vi "AFM_OverlayConfigurator.vi"(8 "Error In":errorcluster, 9 "Image Data Range (Main)":cluster{dbl, dbl}(slide)={46.98275862068965, 0.0} scale=0.0..100.0, 11 "Main Image (IBW)":path) -> (0 "Error Out":errorcluster)   [LabVIEW 2019]
uses:
  <vilib>/vision/Image Controls.llb/IMAQ Image.ctl
  <vilib>/JDP Science/JSONtext/JSONtext.lvlib
panel:
  out "Background out":T1
  in  "Tab Control":enum32{"App", "Documentation"}(tab)
  in  "Load Images":bool
  in  "Exit":bool
  in  "Overlay Image (IBW)":path
  out "Inkscape Config":T2 {"Width/Height" format="%#_6p"; "Y Pos" format="%#_6p"; "X Pos" format="%#_6p"}
  out "Render (Main)":T1(plugin-control)
  in  "Save Overlay":bool
  out "Render (Overlay)":T1(plugin-control)
  in  "Image Data Range (Overlay)":cluster{dbl, dbl}(slide)={46.98275862068965, 0.0} scale=0.0..100.0
  # "AFM Image Overlay Configurator"
  # "This program helps you to overlay/align two AFM background images in Inkscape. Usually this is used when the user needs to overlay a smaller HighRes scan with a \nLarger LowRes scan in Inkscape to design their devices with reference to a smaller feature on the sample.\n\nOperation:\n1. Open the path of your Main Scan (IBW)\n2. Open the path of your Reference (Overlay) Image (IBW)\n3. Click Load- This will:\n         i) Give you a preview of the two images\n         ii) Give you the Inkscape Parameters of the Overlay\n\n4. Adjust the sliders to get a clear enough image\n5. Click 'Save Overlay as JPG' to save a JPG copy of your overlay\n6. Import/DragnDrop the JPG to your Main Inkscape file and input the calculated Inkscape Params for the overlay image\n\n\n\n\n\n\n\n\n\n\n\n\n\n\n\n\nAuthored by Pubudu W."
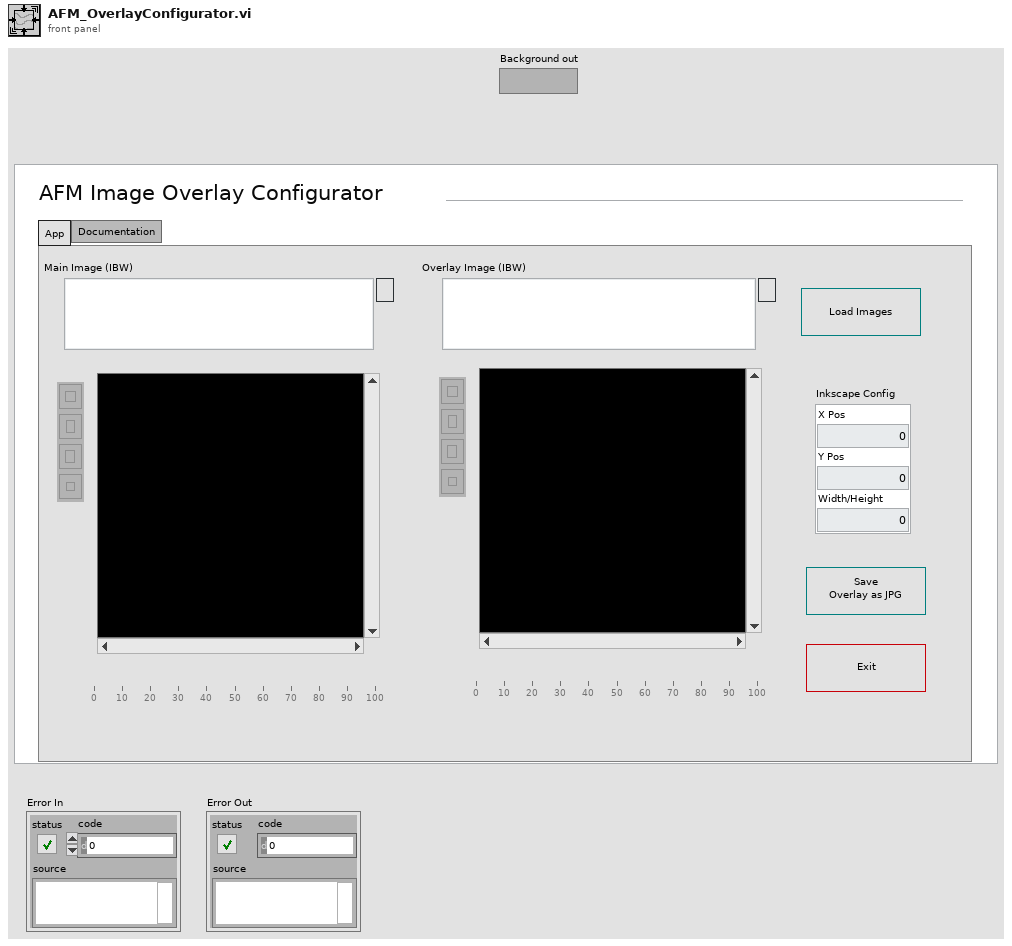
[diagram p1: front panel]
types:
  T1 = typedef "IMAQ Image.ctl" = refnum<image>
  T2 = cluster{"X Pos":dbl, "Y Pos":dbl, "Width/Height":dbl}
  T3 = enum32{"Invalid", "Standard", "Closed", "Hidden", "Minimized", "Maximized"}
  T4 = enum32{"invalid app kind", "Development System", "Run Time System", "Student Edition", "Embedded LabVIEW", "Evaluation", "Custom"}
  T5 = cluster{"Core":cluster{"Current VI Reference":refnum<vi>, "Close Panel on Exit?":bool}, "Main Image Params":cluster{"Initial ScanSize":string, "Initial XOffset":string, "Initial YOffset":string}, "Overlay Image Params":cluster{"Initial ScanSize":string, "Initial XOffset":string, "Initial YOffset":string}}
  T6 = cluster{"Initial ScanSize":string, "Initial XOffset":string, "Initial YOffset":string}
  T7 = cluster{"Current VI Reference":refnum<vi>, "Close Panel on Exit?":bool}
  T8 = typedef "Image Type" = u32
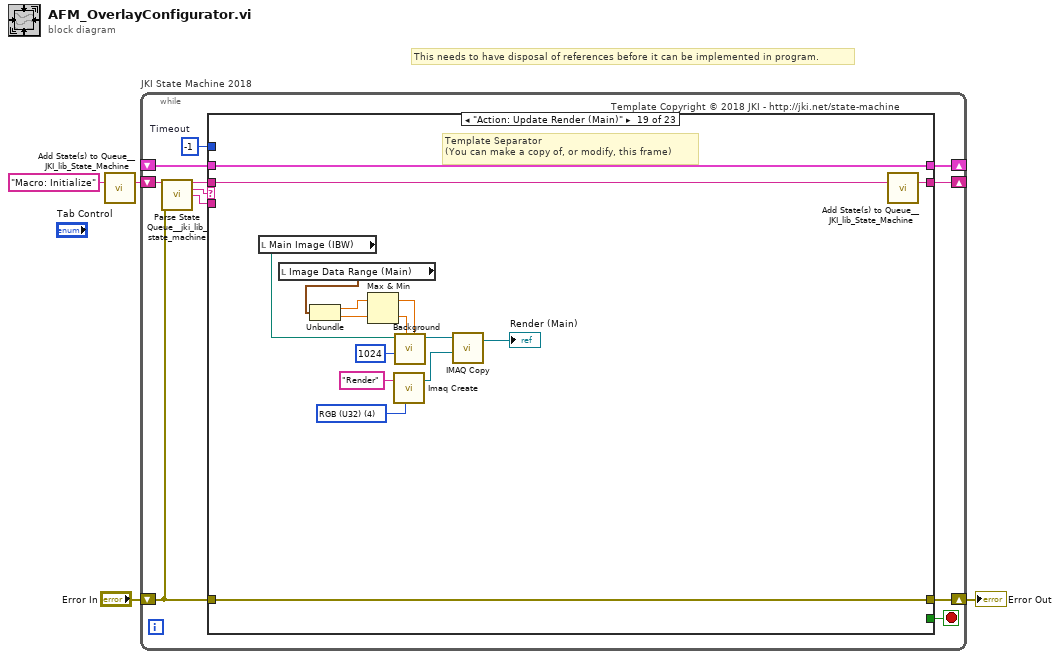
[diagram p0: block diagram]
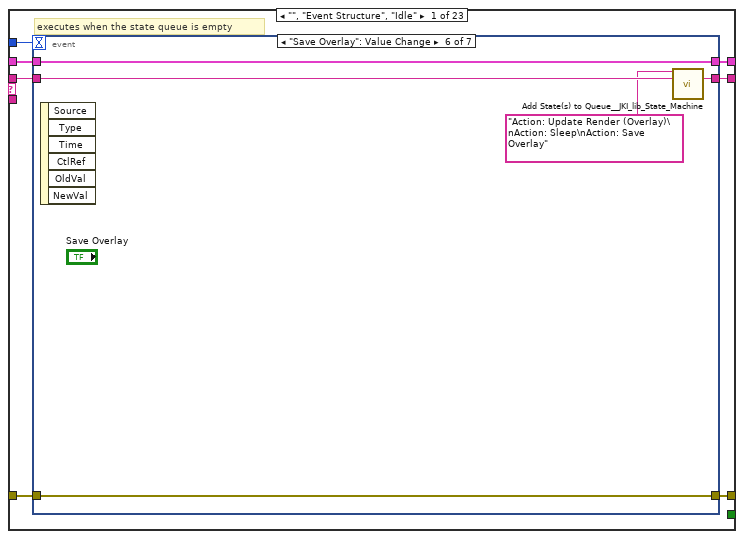
[diagram p2: hidden frame]
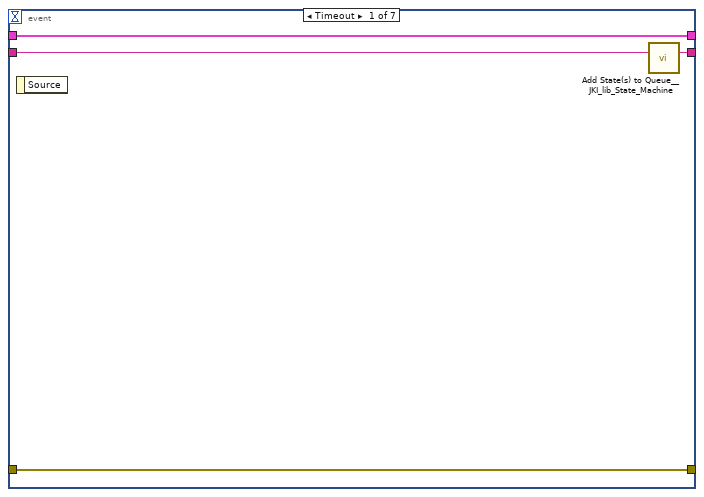
[diagram p3: hidden frame]
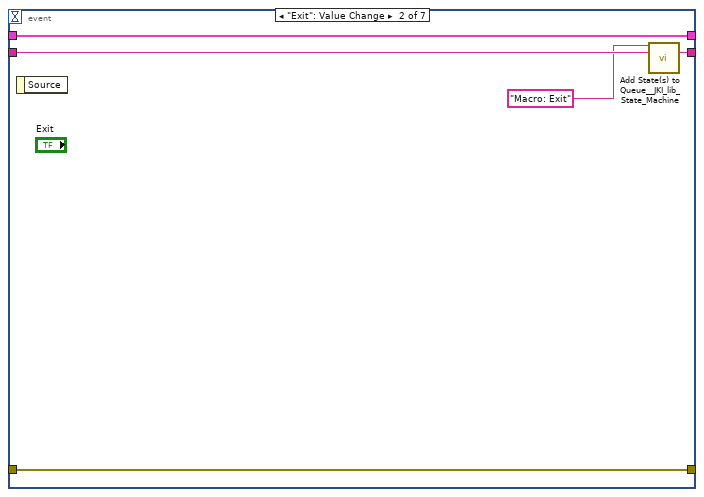
[diagram p4: hidden frame]
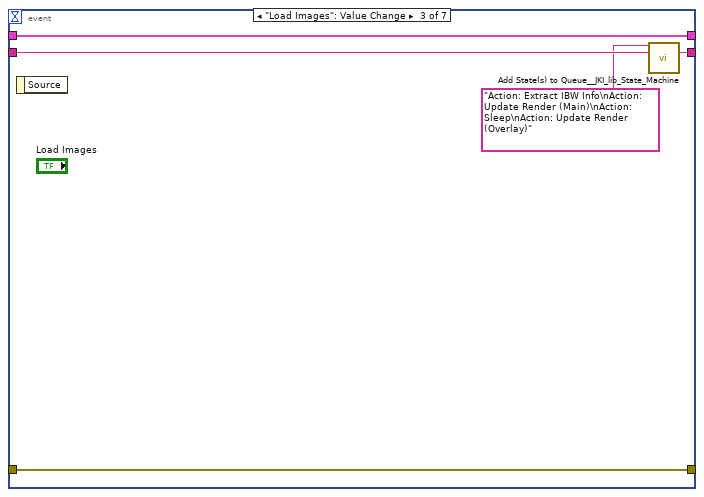
[diagram p5: hidden frame]
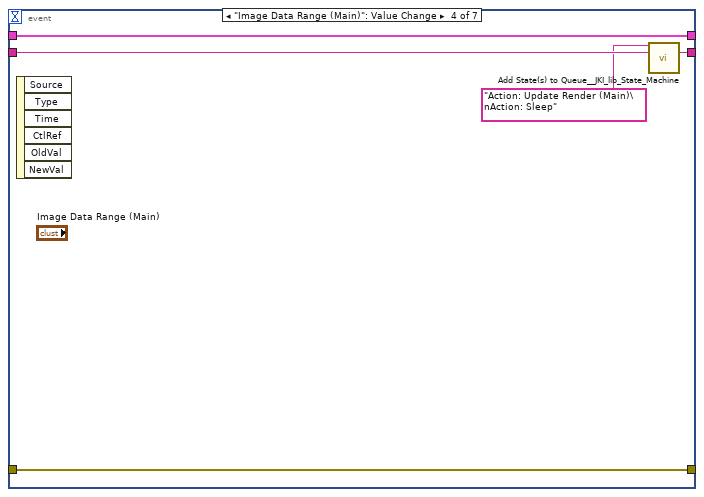
[diagram p6: hidden frame]
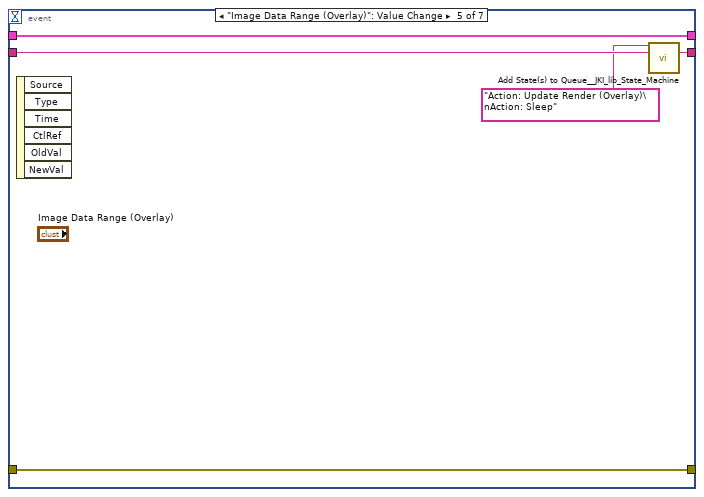
[diagram p7: hidden frame]
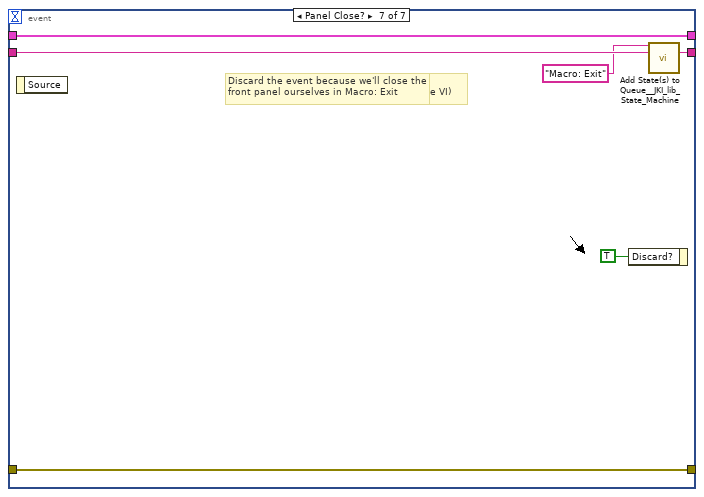
[diagram p8: hidden frame]
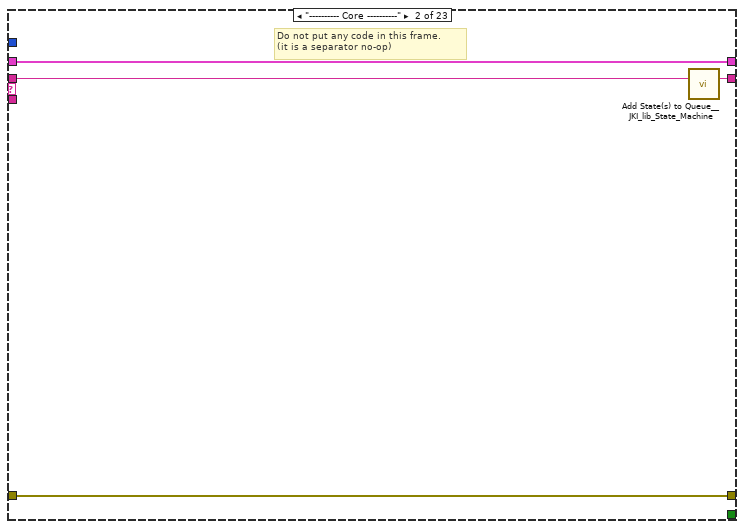
[diagram p9: hidden frame]
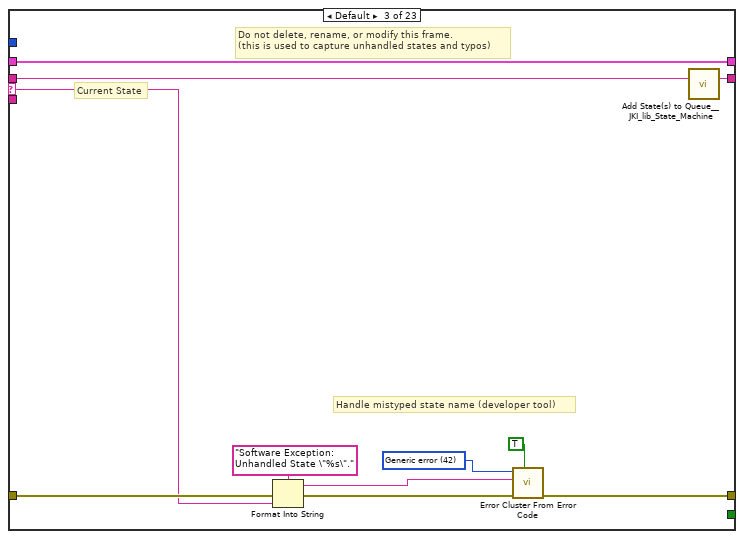
[diagram p10: hidden frame]
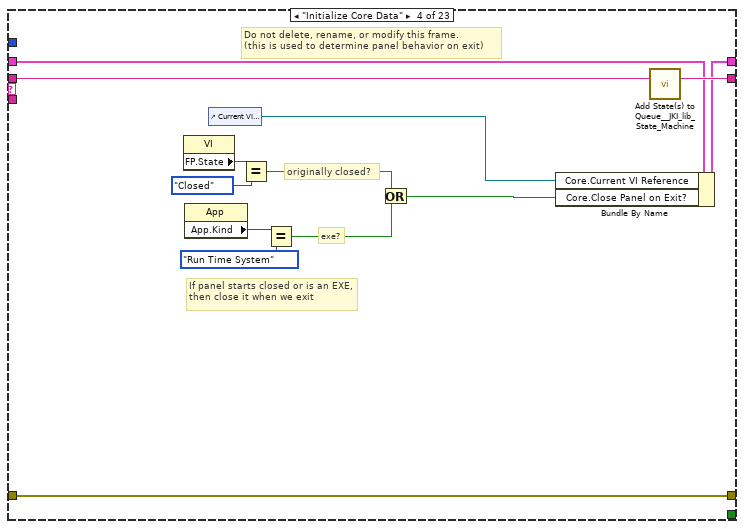
[diagram p11: hidden frame]
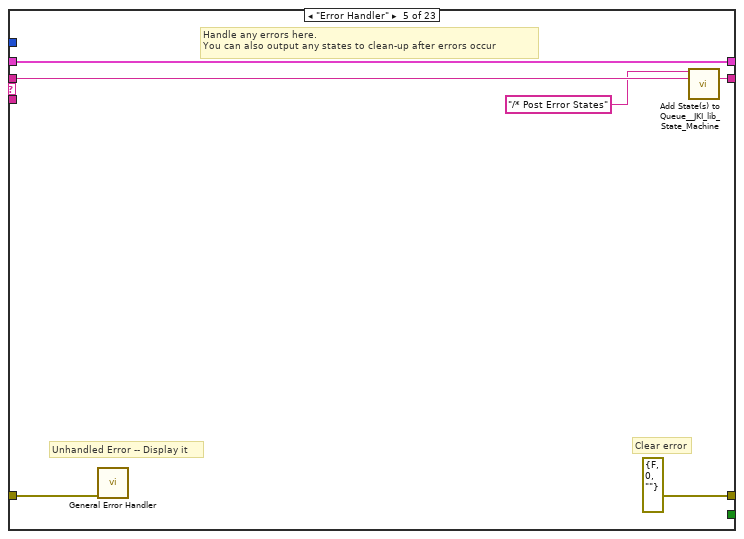
[diagram p12: hidden frame]
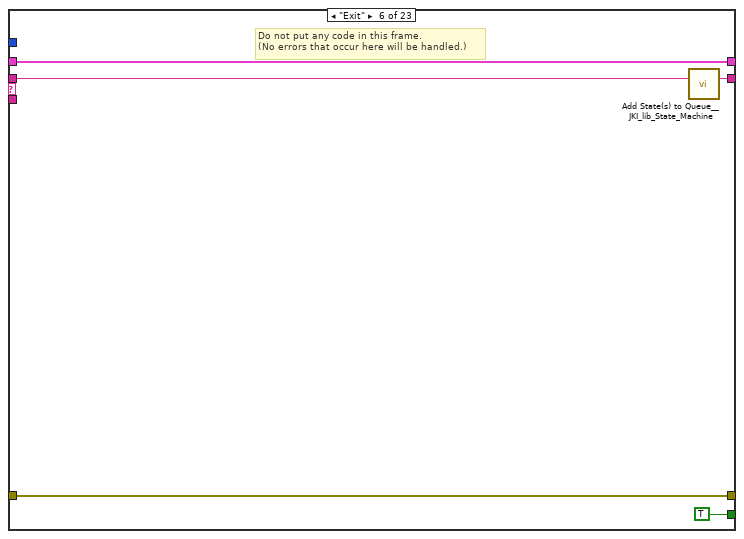
[diagram p13: hidden frame]
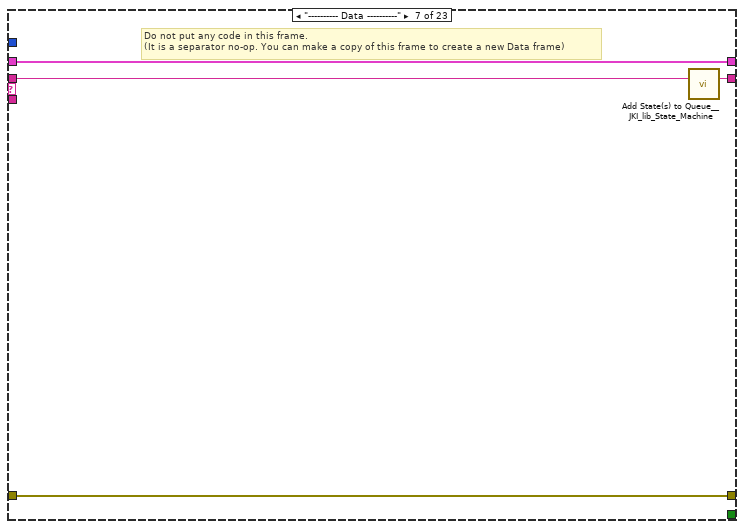
[diagram p14: hidden frame]
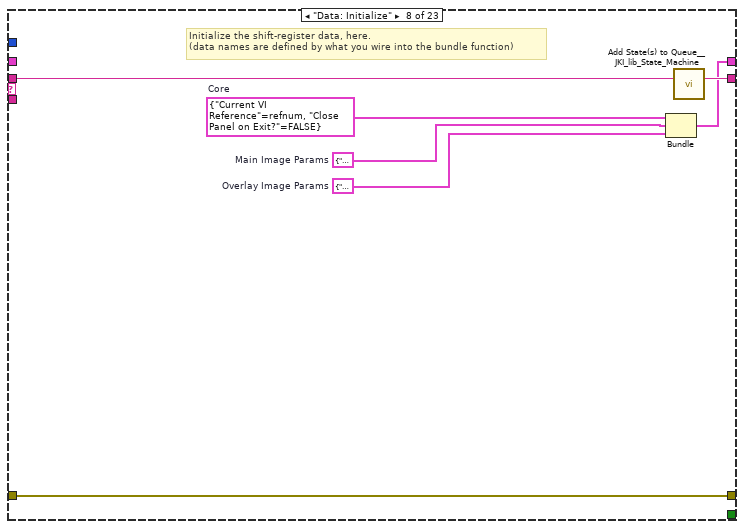
[diagram p15: hidden frame]
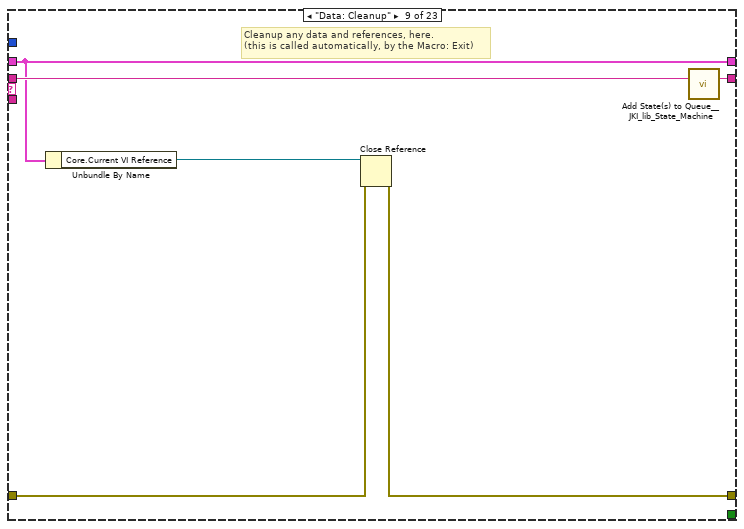
[diagram p16: hidden frame]
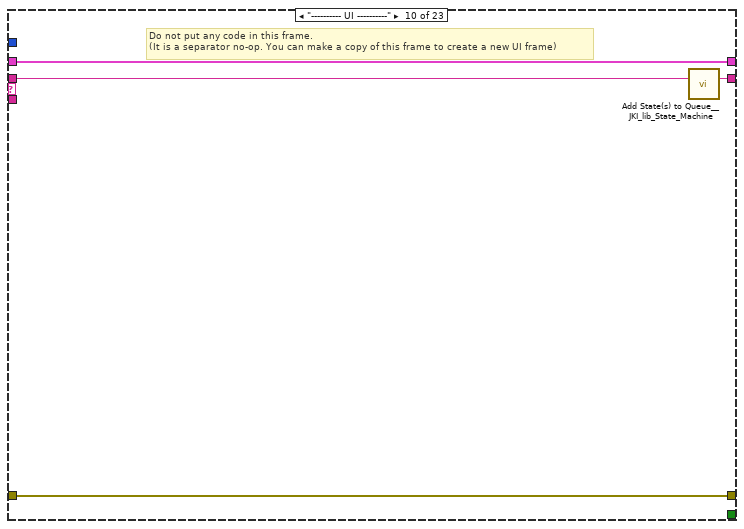
[diagram p17: hidden frame]
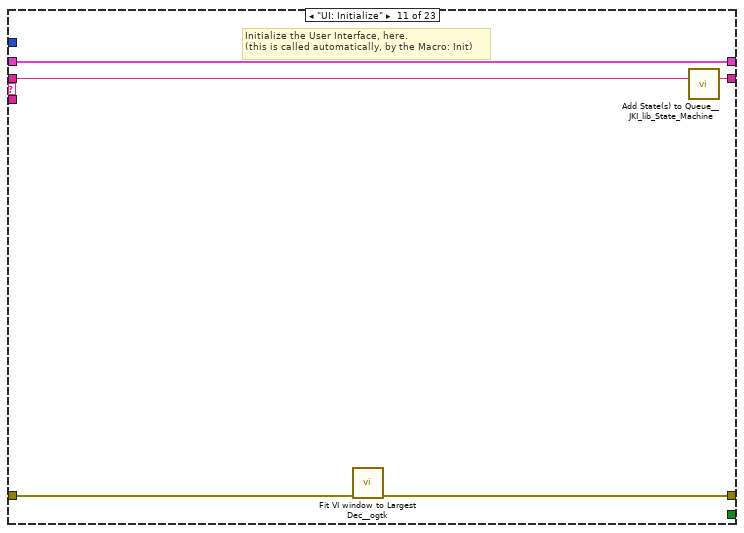
[diagram p18: hidden frame]
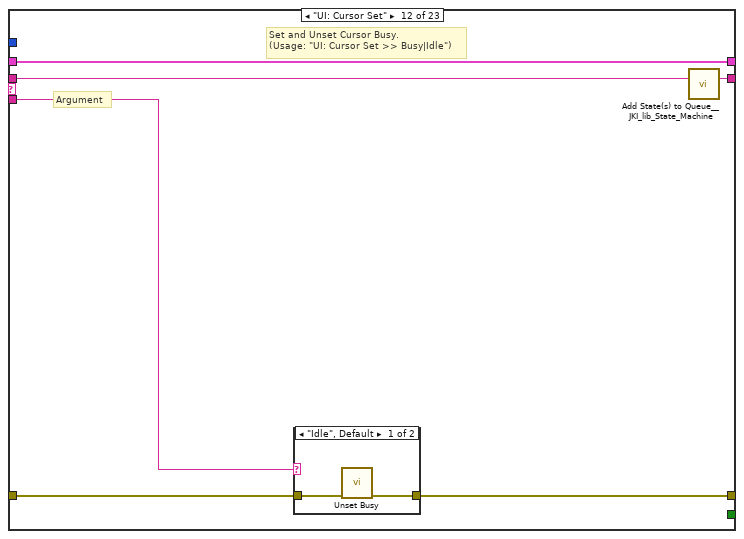
[diagram p19: hidden frame]
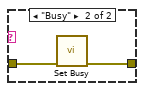
[diagram p20: hidden frame]
diagram:
  # "This needs to have disposal of references before it can be implemented in program."
  n1 = call <vilib>:"Add State(s) to Queue__JKI_lib_State_Machine.vi"("State(s) in (\"\")"="Macro: Initialize") -> ("States Out"=w4:string)  [unwired: 14 in]
  n2 = while "JKI State Machine 2018" {
    shift-right: [w8] -> _
    shift-left: _ -> [w7]
    shift-right: [w11] -> w1
    shift-left: "Error In" -> [w5]
    shift-right: [w10] -> _
    shift-left: w4 -> [w12]
    stop <- w9 stop-if-true
    w6 = -1  # Timeout
    # "Template Copyright © 2018 JKI - http://jki.net/state-machine"
    n3 = call <vilib>:"Parse State Queue__jki_lib_state_machine.vi"("State Queue"=w12, "Error In (no error)"=w5) -> ("Remaining States"=w14:string, "Current State"=w15:string, "Arguments"=w13:string)  [unwired: 11 in]
    n4 = case shown="\"Action: Update Render (Main)\"" w15 {
      selector: w15 -> [_ _ w62 _ _ _ _ _ _ _ _ _ _ _ _ _ _ _ _ _ _ _ _]
      tunnel: w14 -> [w22 w61 w66 w85 w91 w96 w100 w107 w113 w117 w122 w128 w139 w208 w213 w223 w227 w246 w262 w278 w284 w297 w324]
      tunnel: w13 -> [_ _ _ _ _ _ _ _ _ _ _ w123 w133 _ _ _ _ _ _ _ _ _ _]
      tunnel: w7 -> [w20 w58 w64 w78 w88 w94 w97 _ w108 w114 w120 w126 w135 w205 w210 w220 w224 w233 w259 w275 w282 w295 w321]
      tunnel: [w19 w59 w68 w82 errorcluster {"status"=FALSE, "code"=0, "source"=""} ("error out") w93 w98 w104 w109 w115 w119 w124 w136 w206 w211 w221 w225 w235 w260 w276 w279 w285 w322] -> w11
      tunnel: w5 -> [w18 w59 w67 w82 w87 w93 w98 w104 w110 w115 w118 w125 w137 w206 w211 w221 w225 w243 w260 w276 w280 w287 w322]
      tunnel: [w21 w60 w65 w84 w90 w95 w99 w106 w112 w116 w121 w127 w138 w207 w212 w222 w226 w245 w261 w277 w283 w296 w323] -> w10
      tunnel: [_ _ _ _ _ TRUE _ _ _ _ _ _ _ _ _ _ _ _ _ _ _ _ _] -> w9
      tunnel: [w17 w58 w64 w83 w88 w94 w97 w105 w108 w114 w120 w126 w135 w205 w210 w220 w224 w232 w259 w275 w282 w295 w321] -> w8
      tunnel: w6 -> [w16 _ _ _ _ _ _ _ _ _ _ _ _ _ _ _ _ _ _ _ _ _ _]
      frame "", "Event Structure", "Idle" {
        # "executes when the state queue is empty"
        n5 = event shown="[5] \"Save Overlay\": Value Change" {
          selector: _ -> [_ _ _ _ _ _ _]
          dyn-events: _ -> [_ _ _ _ _ _ _]
          timeout: w16 -> [_ _ _ _ _ _ _]
          tunnel: w22 -> [w26 w31 w36 w41 w46 w51 w57]
          tunnel: [w25 w30 w35 w40 w45 w50 w56] -> w21
          tunnel: w20 -> [w23 w28 w33 w38 w43 w48 w54]
          tunnel: [w24 w29 w34 w39 w44 w49 w55] -> w19
          tunnel: w18 -> [w24 w29 w34 w39 w44 w49 w55]
          tunnel: [w23 w28 w33 w38 w43 w48 w54] -> w17
          event Timeout {
            n6 = event-data() -> ()  [unwired: 1 in, 1 out]
            n7 = call <vilib>:"Add State(s) to Queue__JKI_lib_State_Machine.vi"("State(s) in (\"\")"=w26) -> ("States Out"=w25:string)  [unwired: 14 in]
          }
          event "Exit": Value Change {
            n8 = event-data() -> ()  [unwired: 1 in, 1 out]
            n9 = call <vilib>:"Add State(s) to Queue__JKI_lib_State_Machine.vi"("State(s) in Front (\"\")"="Macro: Exit", "State(s) in (\"\")"=w31) -> ("States Out"=w30:string)  [unwired: 13 in]
          }
          event "Load Images": Value Change {
            n10 = event-data() -> ()  [unwired: 1 in, 1 out]
            n11 = call <vilib>:"Add State(s) to Queue__JKI_lib_State_Machine.vi"("State(s) in Front (\"\")"="Action: Extract IBW Info\nAction: Update Render (Main)\nAction: Sleep\nAction: Update Render (Overlay)", "State(s) in (\"\")"=w36) -> ("States Out"=w35:string)  [unwired: 13 in]
          }
          event "Image Data Range (Main)": Value Change {
            n12 = event-data() -> ()  [unwired: 1 in, 6 out]
            n13 = call <vilib>:"Add State(s) to Queue__JKI_lib_State_Machine.vi"("State(s) in Front (\"\")"="Action: Update Render (Main)\nAction: Sleep", "State(s) in (\"\")"=w41) -> ("States Out"=w40:string)  [unwired: 13 in]
          }
          event "Image Data Range (Overlay)": Value Change {
            n14 = event-data() -> ()  [unwired: 1 in, 6 out]
            n15 = call <vilib>:"Add State(s) to Queue__JKI_lib_State_Machine.vi"("State(s) in Front (\"\")"="Action: Update Render (Overlay)\nAction: Sleep", "State(s) in (\"\")"=w46) -> ("States Out"=w45:string)  [unwired: 13 in]
          }
          event "Save Overlay": Value Change {
            n16 = event-data() -> ()  [unwired: 1 in, 6 out]
            n17 = call <vilib>:"Add State(s) to Queue__JKI_lib_State_Machine.vi"("State(s) in Front (\"\")"="Action: Update Render (Overlay)\nAction: Sleep\nAction: Save Overlay", "State(s) in (\"\")"=w51) -> ("States Out"=w50:string)  [unwired: 13 in]
          }
          event Panel Close? {
            # "Discard the event because we'll close the front panel ourselves in Macro: Exit"
            # "Close Panel button (pressed) Event\n(this executes Macro: Exit to terminate the VI)"
            n18 = event-data() -> ()  [unwired: 1 in, 1 out]
            n19 = event-data("Discard?"=TRUE) -> ()  [unwired: 1 in, 1 out]
            n20 = call <vilib>:"Add State(s) to Queue__JKI_lib_State_Machine.vi"("State(s) in Front (\"\")"="Macro: Exit", "State(s) in (\"\")"=w57) -> ("States Out"=w56:string)  [unwired: 13 in]
          }
        }
      }
      frame "---------- Core ----------" {
        # "Do not put any code in this frame.\n(it is a separator no-op)"
        n21 = call <vilib>:"Add State(s) to Queue__JKI_lib_State_Machine.vi"("State(s) in (\"\")"=w61) -> ("States Out"=w60:string)  [unwired: 14 in]
      }
      frame Default {
        w71 = 42 items=["No error", "Argument error", "Memory is full", "Out of zone", "End of file", "File already open", "Generic file I/O error", "File not found", "File permission error", "Disk is full", "Duplicate path", "Too many files open", "System feature not enabled", "Resource file not found", "Cannot add resource", "Resource not found", "Image not found", "Image memory error", "Pen does not exist", "Config type invalid", "Config token not found", "Config parse error", "Config memory error", "Bad external code format", "Bad external code offset", "External code not present", "Null window", "Destroy window error", "Null menu", "Print aborted", "Bad print record", "Print driver error", "Windows error during printing", "Memory error during printing", "Print dialog error", "Generic print error", "Invalid device refnum", "Device not found", "Device parameter error", "Device unit error", "Cannot open device", "Device call aborted", "Generic error", "Cancelled by user", "Object ID too low", "Object ID too high", "Object not in heap", "Unknown heap", "Unknown object (invalid DefProc)", "Unknown object (DefProc not in table)", "Message out of range", "Invalid (null) method", "Unknown message", "Manager call not supported", "Bad address", "Network operation in progress", "Network operation timed out", "Connection is busy", "Network attribute not supported", "Network error", "Address in use", "System out of memory", "Connection aborted", "Connection refused", "Not connected", "Already connected", "Connection closed", "Initialization error (interapplication manager)", "Bad occurrence", "Wait on unbound occurrence handler", "Occurrence queue overflow", "Datalog type conflict", "Unused", "Unrecognized type (interapplication manager)", "Memory corrupt", "Failed to make temporary DLL", "Old CIN version", "Drag socket not found", "Failed to load drop-object", "Failed to register OLE object", "Failed to release OLE object", "Format specifier type mismatch", "Unknown format specifier", "Too few format specifiers", "Too many format specifiers", "Scan failed", "Newer CIN version", "Error converting to variant", "Runtime menu error", "Password tampered", "Variant attribute not found", "Incompatible variant data type", "Event data is not available", "Event Store is not present", "Occurrence is not found", "Event Queue is not created", "Event info is not available", "Refnum passed is NULL", "Error retrieving Class GUID", "Error retrieving CoClass GUID", "Error retrieving TypeLib GUID.", "Bad built application magic bytes.", "Specific driver is different from the specific driver associated with the Logical Name.", "There is no session opened to the class driver.", "Max Error", "MAX - Error with config objects", "MAX - Error loading configuration", "MAX - Group not supported"]
        # "Current State"
        # "Do not delete, rename, or modify this frame.\n(this is used to capture unhandled states and typos)"
        # "Handle mistyped state name (developer tool)"
        n22 = Format Into String(format string="Software Exception: Unhandled State \"%s\"." ("message"), error in=w67, w62) -> (resulting string=w70:string, error out=w69:errorcluster)  [unwired: 1 in]
        n23 = call <vilib>:"Error Cluster From Error Code.vi"("show call chain? (False)"=TRUE, "error in (no error)"=w69, "error message (\"\")"=w70, "error code (0)"=w71) -> ("error out"=w68:errorcluster)  [unwired: 5 in]
        n24 = call <vilib>:"Add State(s) to Queue__JKI_lib_State_Machine.vi"("State(s) in (\"\")"=w66) -> ("States Out"=w65:string)  [unwired: 14 in]
      }
      frame "Initialize Core Data" {
        # "Do not delete, rename, or modify this frame.\n(this is used to determine panel behavior on exit)"
        # "originally closed?"
        # "exe?"
        # "If panel starts closed or is an EXE, then close it when we exit"
        n25 = property class="VI"() -> ("FP.State"=w75:T3)  [unwired: 2 in, 2 out]
        n26 = property class="App"() -> ("App.Kind"=w81:T4)  [unwired: 2 in, 2 out]
        n27 = control-ref of="Current VI Reference"() -> (w76:refnum<vi>)
        n28 = Equal?(x=w75, y=T3."Closed" ("Front Panel Window:State")) -> (x = y?=w73:bool)
        n29 = Equal?(x=w81, y=T4."Run Time System" ("Application:Kind")) -> (x = y?=w79:bool)
        n30 = Or(x=w73, y=w79) -> (x .or. y?=w77:bool)
        n31 = Bundle By Name(cluster=w78, "Core.Current VI Reference"=w76, "Core.Close Panel on Exit?"=w77) -> (w83:T5)
        n32 = call <vilib>:"Add State(s) to Queue__JKI_lib_State_Machine.vi"("State(s) in (\"\")"=w85) -> ("States Out"=w84:string)  [unwired: 14 in]
      }
      frame "Error Handler" {
        # "Unhandled Error -- Display it"
        # "Handle any errors here.\nYou can also output any states to clean-up after errors occur"
        # "Clear error"
        n33 = call <vilib>:"General Error Handler.vi"("error in (no error)"=w87) -> ()  [unwired: 10 in, 5 out]
        n34 = call <vilib>:"Add State(s) to Queue__JKI_lib_State_Machine.vi"("State(s) in Front (\"\")"="/* Post Error States", "State(s) in (\"\")"=w91) -> ("States Out"=w90:string)  [unwired: 13 in]
      }
      frame "Exit" {
        # "Do not put any code in this frame.\n(No errors that occur here will be handled.)"
        n35 = call <vilib>:"Add State(s) to Queue__JKI_lib_State_Machine.vi"("State(s) in (\"\")"=w96) -> ("States Out"=w95:string)  [unwired: 14 in]
      }
      frame "---------- Data ----------" {
        # "Do not put any code in this frame.\n(It is a separator no-op. You can make a copy of this frame to create a new Data frame)"
        n36 = call <vilib>:"Add State(s) to Queue__JKI_lib_State_Machine.vi"("State(s) in (\"\")"=w100) -> ("States Out"=w99:string)  [unwired: 14 in]
      }
      frame "Data: Initialize" {
        w101 = T6 {"Initial ScanSize"="", "Initial XOffset"="", "Initial YOffset"=""}  # Overlay Image Params
        w102 = T6 {"Initial ScanSize"="", "Initial XOffset"="", "Initial YOffset"=""}  # Main Image Params
        w103 = T7 {"Current VI Reference"=refnum, "Close Panel on Exit?"=FALSE}  # Core
        # "Initialize the shift-register data, here.\n(data names are defined by what you wire into the bundle function)"
        n37 = Bundle("Core"=w103, "Main Image Params"=w102, "Overlay Image Params"=w101) -> (w105:T5)  [unwired: 1 in]
        n38 = call <vilib>:"Add State(s) to Queue__JKI_lib_State_Machine.vi"("State(s) in (\"\")"=w107) -> ("States Out"=w106:string)  [unwired: 14 in]
      }
      frame "Data: Cleanup" {
        # "Cleanup any data and references, here.\n(this is called automatically, by the Macro: Exit)"
        n39 = Unbundle By Name(w108) -> ("Core.Current VI Reference"=w111:refnum<vi>)
        n40 = Close Reference(reference=w111, error in (no error)=w110) -> (error out=w109:errorcluster)
        n41 = call <vilib>:"Add State(s) to Queue__JKI_lib_State_Machine.vi"("State(s) in (\"\")"=w113) -> ("States Out"=w112:string)  [unwired: 14 in]
      }
      frame "---------- UI ----------" {
        # "Do not put any code in this frame.\n(It is a separator no-op. You can make a copy of this frame to create a new UI frame)"
        n42 = call <vilib>:"Add State(s) to Queue__JKI_lib_State_Machine.vi"("State(s) in (\"\")"=w117) -> ("States Out"=w116:string)  [unwired: 14 in]
      }
      frame "UI: Initialize" {
        # "Initialize the User Interface, here.\n(this is called automatically, by the Macro: Init)"
        n43 = call <userlib>:"Fit VI window to Largest Dec__ogtk.vi"("error in (no error)"=w118) -> ("error out"=w119:errorcluster)  [unwired: 5 in, 1 out]
        n44 = call <vilib>:"Add State(s) to Queue__JKI_lib_State_Machine.vi"("State(s) in (\"\")"=w122) -> ("States Out"=w121:string)  [unwired: 14 in]
      }
      frame "UI: Cursor Set" {
        # "Argument"
        # "Set and Unset Cursor Busy.\n(Usage: \"UI: Cursor Set >> Busy|Idle\")"
        n45 = case shown="\"Idle\", Default" w123 {
          tunnel: w125 -> [w130 w132]
          tunnel: [w129 w131] -> w124
          frame "Idle", Default {
            n46 = call <vilib>:"Unset Busy.vi"("error in (no error)"=w130) -> ("error out"=w129:errorcluster)  [unwired: 10 in]
          }
          frame "Busy" {
            n47 = call <vilib>:"Set Busy.vi"("error in (no error)"=w132) -> ("error out"=w131:errorcluster)  [unwired: 9 in, 1 out]
          }
        }
        n48 = call <vilib>:"Add State(s) to Queue__JKI_lib_State_Machine.vi"("State(s) in (\"\")"=w128) -> ("States Out"=w127:string)  [unwired: 14 in]
      }
      frame "UI: Front Panel State" {
        # "Argument"
        # "Set Front Panel Open or Closed\n(Usage: \"UI: Front Panel State >> Open|Close\")"
        n49 = Unbundle By Name(w135) -> ("Core.Current VI Reference"=w134:refnum<vi>)
        n50 = case shown="\"Open\", \"Standard\", Default" w133 {
          tunnel: w137 -> [w145 w160 w171 w184 w197]
          tunnel: [w147 w161 w173 w186 w199] -> w136
          tunnel: w134 -> [w146 w158 w172 w185 w198]
          frame "Open", "Standard", Default {
            w140 = T3."Standard" ("State")
            n51 = property class="VI"(reference=w146, error in=w145) -> (reference out=w143:refnum<vi>, error out=w144:errorcluster, "FP.State"=w142:T3)
            n52 = Not Equal?(x=w142, y=w140) -> (x != y?=w141:bool)
            n53 = case shown="True" w141 {
              tunnel: [w151 w153] -> w147
              tunnel: w144 -> [w150 w153]
              tunnel: w143 -> [w149 _]
              tunnel: w140 -> [w148 _]
              frame True {
                n54 = invoke class="VI" method="FP.Open"(reference=w149, error in=w150, "Activate"=TRUE, "State"=w148) -> (error out=w151:errorcluster)  [unwired: 1 in, 4 out]
              }
              frame False {
              }
            }
          }
          frame "Close", "Closed" {
            n55 = property class="VI"(reference=w158, error in=w160) -> (reference out=w157:refnum<vi>, error out=w159:errorcluster, "FP.State"=w155:T3)
            n56 = Not Equal?(x=w155, y=T3."Closed" ("Front Panel Window:State")) -> (x != y?=w154:bool)
            n57 = case shown="True" w154 {
              tunnel: [w162 w165] -> w161
              tunnel: w159 -> [w162 w164]
              tunnel: w157 -> [_ w163]
              frame False {
              }
              frame True {
                n58 = invoke class="VI" method="FP.Close"(reference=w163, error in=w164) -> (error out=w165:errorcluster)  [unwired: 1 in, 2 out]
              }
            }
          }
          frame "Hidden", "Hide" {
            w166 = T3."Hidden" ("State")
            n59 = property class="VI"(reference=w172, error in=w171) -> (reference out=w169:refnum<vi>, error out=w170:errorcluster, "FP.State"=w168:T3)
            n60 = Not Equal?(x=w168, y=w166) -> (x != y?=w167:bool)
            n61 = case shown="True" w167 {
              tunnel: [w177 w178] -> w173
              tunnel: w170 -> [w176 w178]
              tunnel: w169 -> [w175 _]
              tunnel: w166 -> [w174 _]
              frame True {
                n62 = invoke class="VI" method="FP.Open"(reference=w175, error in=w176, "State"=w174) -> (error out=w177:errorcluster)  [unwired: 2 in, 4 out]
              }
              frame False {
              }
            }
          }
          frame "Minimize", "Minimized" {
            w179 = T3."Minimized" ("State")
            n63 = property class="VI"(reference=w185, error in=w184) -> (reference out=w182:refnum<vi>, error out=w183:errorcluster, "FP.State"=w181:T3)
            n64 = Not Equal?(x=w181, y=w179) -> (x != y?=w180:bool)
            n65 = case shown="True" w180 {
              tunnel: [w190 w191] -> w186
              tunnel: w183 -> [w189 w191]
              tunnel: w182 -> [w188 _]
              tunnel: w179 -> [w187 _]
              frame True {
                n66 = invoke class="VI" method="FP.Open"(reference=w188, error in=w189, "State"=w187) -> (error out=w190:errorcluster)  [unwired: 2 in, 4 out]
              }
              frame False {
              }
            }
          }
          frame "Maximize", "Maximized" {
            w192 = T3."Maximized" ("State")
            n67 = property class="VI"(reference=w198, error in=w197) -> (reference out=w195:refnum<vi>, error out=w196:errorcluster, "FP.State"=w194:T3)
            n68 = Not Equal?(x=w194, y=w192) -> (x != y?=w193:bool)
            n69 = case shown="True" w193 {
              tunnel: [w203 w204] -> w199
              tunnel: w196 -> [w202 w204]
              tunnel: w195 -> [w201 _]
              tunnel: w192 -> [w200 _]
              frame True {
                n70 = invoke class="VI" method="FP.Open"(reference=w201, error in=w202, "State"=w200) -> (error out=w203:errorcluster)  [unwired: 2 in, 4 out]
              }
              frame False {
              }
            }
          }
        }
        n71 = call <vilib>:"Add State(s) to Queue__JKI_lib_State_Machine.vi"("State(s) in (\"\")"=w139) -> ("States Out"=w138:string)  [unwired: 14 in]
      }
      frame "---------- Macro ----------" {
        # "Do not put any code in this frame.\n(It is a separator no-op. You can make a copy of this frame to create a new Macro frame)"
        n72 = call <vilib>:"Add State(s) to Queue__JKI_lib_State_Machine.vi"("State(s) in (\"\")"=w208) -> ("States Out"=w207:string)  [unwired: 14 in]
      }
      frame "Macro: Initialize" {
        w209 = "Data: Initialize\nInitialize Core Data\nUI: Initialize\nUI: Front Panel State >> Open"  # Data: Initialize Initialize Core Data UI: Initialize UI: Front Panel State >> Open
        # "Initialization Macro\n(This is called once, when the VI starts)"
        n73 = call <vilib>:"Add State(s) to Queue__JKI_lib_State_Machine.vi"("State(s) in Front (\"\")"=w209, "State(s) in (\"\")"=w213) -> ("States Out"=w212:string)  [unwired: 13 in]
      }
      frame "Macro: Exit" {
        # "Exit Macro\n(This is called once, when the VI exits)"
        n74 = Unbundle By Name(w220) -> ("Core.Close Panel on Exit?"=w219:bool)
        n75 = Select(t="UI: Front Panel State >> Close", s=w219, f="") -> (s? t:f=w216:string)
        n76 = call <vilib>:"Add State(s) to Queue__JKI_lib_State_Machine.vi"("State(s) in (\"\")"=w216, "State(s) at Back (\"\")"="Data: Cleanup\nExit") -> ("States Out"=w214:string)  [unwired: 13 in]
        n77 = call <vilib>:"Add State(s) to Queue__JKI_lib_State_Machine.vi"("State(s) in Front (\"\")"=w214, "State(s) in (\"\")"=w223) -> ("States Out"=w222:string)  [unwired: 13 in]
      }
      frame "---------- Action ----------" {
        # "Template Separator\n(You can make a copy of, or modify, this frame)"
        n78 = call <vilib>:"Add State(s) to Queue__JKI_lib_State_Machine.vi"("State(s) in (\"\")"=w227) -> ("States Out"=w226:string)  [unwired: 14 in]
      }
      frame "Action: Extract IBW Info" {
        w234 = T6 {"Initial ScanSize"="", "Initial XOffset"="", "Initial YOffset"=""}
        # "Your code here.\n(You can make a copy of, or modify, this frame)"
        n79 = call "Read IBW File.vi"("error in (no error)"=w243, "Path"="Main Image (IBW)") -> ("error out"=w241:errorcluster, "Notes LUT"=w242:variant)  [unwired: 7 in, 1 out]
        n80 = call <vilib>:"Variant to JSON Text.vi"("error in (no error)"=w241, "Variant"=w242) -> ("<JSON>"=w238:string)  [unwired: 7 in, 2 out]
        n81 = Unflatten From JSON(JSON string=w238, type and defaults=w234) -> (value=w230:T6)  [unwired: 5 in, 1 out]
        n82 = call "Read IBW File.vi"("Path"="Overlay Image (IBW)") -> ("error out"=w239:errorcluster, "Notes LUT"=w240:variant)  [unwired: 8 in, 1 out]
        n83 = call <vilib>:"Variant to JSON Text.vi"("error in (no error)"=w239, "Variant"=w240) -> ("error out"=w236:errorcluster, "<JSON>"=w237:string)  [unwired: 7 in, 1 out]
        n84 = Unflatten From JSON(JSON string=w237, type and defaults=w234, error in (no error)=w236) -> (value=w231:T6, error out=w235:errorcluster)  [unwired: 4 in]
        n85 = Bundle By Name(cluster=w233, "Main Image Params"=w230, "Overlay Image Params"=w231) -> (w232:T5)
        n86 = call <vilib>:"Add State(s) to Queue__JKI_lib_State_Machine.vi"("State(s) in Front (\"\")"="Action: Derive Inkscape Params" ("State(s) in Front (\"\")"), "State(s) in (\"\")"=w246) -> ("States Out"=w245:string)  [unwired: 13 in]
      }
      frame "Action: Update Render (Main)" {
        w253 = T8 4 items=["Grayscale (U8)", "Grayscale (I16)", "Grayscale (SGL)", "Complex (CSG)", "RGB (U32)", "HSL (U32)", "RGB (U64)", "Grayscale (U16)"] ("Image Type")
        # "Template Separator\n(You can make a copy of, or modify, this frame)"
        n87 = local read "Main Image (IBW)"() -> (w249:path)
        n88 = local read "Image Data Range (Main)"() -> (w247:cluster{dbl, dbl})
        n89 = Unbundle(w247) -> (w258:dbl, w257:dbl)
        n90 = Max & Min(x=w258, y=w257) -> (max(x,y)=w251:dbl, min(x,y)=w250:dbl)
        n91 = call "Imaq Create"("Image Name"="Render", "Image Type"=w253) -> ("New Image"=w252:T1)  [unwired: 3 in, 1 out]
        n92 = call "Background.vi"("Image data max"=w251, "Image data min"=w250, "Resolution"=1024, "Image File Path"=w249) -> ("Background out"=w255:T1)  [unwired: 4 in, 3 out]
        n93 = call "IMAQ Copy"("Image Dst"=w252, "Image Src"=w255) -> ("Image Dst Out"=→"Render (Main)":T1)  [unwired: 4 in, 1 out]
        n94 = call <vilib>:"Add State(s) to Queue__JKI_lib_State_Machine.vi"("State(s) in (\"\")"=w262) -> ("States Out"=w261:string)  [unwired: 14 in]
      }
      frame "Action: Update Render (Overlay)" {
        w264 = T8 4 items=["Grayscale (U8)", "Grayscale (I16)", "Grayscale (SGL)", "Complex (CSG)", "RGB (U32)", "HSL (U32)", "RGB (U64)", "Grayscale (U16)"] ("Image Type")
        # "Template Separator\n(You can make a copy of, or modify, this frame)"
        n95 = local read "Overlay Image (IBW)"() -> (w268:path)
        n96 = local read "Image Data Range (Overlay)"() -> (w266:cluster{dbl, dbl})
        n97 = Unbundle(w266) -> (w269:dbl, w270:dbl)
        n98 = Max & Min(x=w269, y=w270) -> (max(x,y)=w273:dbl, min(x,y)=w274:dbl)
        n99 = call "Imaq Create"("Image Name"="Render", "Image Type"=w264) -> ("New Image"=w272:T1)  [unwired: 3 in, 1 out]
        n100 = call "Background.vi"("Image data max"=w273, "Image data min"=w274, "Resolution"=1024, "Image File Path"=w268) -> ("Background out"=w271:T1)  [unwired: 4 in, 3 out]
        "Background out" <- w271
        n101 = call "IMAQ Copy"("Image Dst"=w272, "Image Src"=w271) -> ("Image Dst Out"=→"Render (Overlay)":T1)  [unwired: 4 in, 1 out]
        n102 = call <vilib>:"Add State(s) to Queue__JKI_lib_State_Machine.vi"("State(s) in (\"\")"=w278) -> ("States Out"=w277:string)  [unwired: 14 in]
      }
      frame "Action: Sleep" {
        # "Template Separator\n(You can make a copy of, or modify, this frame)"
        n103 = call "Time Delay"("error in (no error)"=w280, "Delay Time (s)"=0.5) -> ("error out"=w279:errorcluster)  [unwired: 9 in]
        n104 = call <vilib>:"Add State(s) to Queue__JKI_lib_State_Machine.vi"("State(s) in (\"\")"=w284) -> ("States Out"=w283:string)  [unwired: 14 in]
      }
      frame "Action: Save Overlay" {
        # "Template Separator\n(You can make a copy of, or modify, this frame)"
        n105 = local read "Overlay Image (IBW)"() -> (w288:path)
        n106 = call <vilib>:"Get File Extension.vi"("error in (no error)"=w287, "file"=w288) -> ("error out"=w286:errorcluster, "filename without extension"=w292:string)  [unwired: 5 in, 3 out]
        n107 = local read "Background out"() -> (w289:T1)
        n108 = Strip Path(path=w288) -> (stripped path=w294:path)  [unwired: 1 out]
        n109 = Concatenate Strings(w292, "_overlay.jpg" ("string")) -> (w290:string)
        n110 = Build Path(base path=w294, name or relative path=w290) -> (appended path=w293:path)
        n111 = call-poly "IMAQ Write File 2"("error in (no error)"=w286, "File Path"=w293, "Image"=w289) -> ("error out"=w285:errorcluster)  [unwired: 7 in, 1 out]
        n112 = call <vilib>:"Add State(s) to Queue__JKI_lib_State_Machine.vi"("State(s) in (\"\")"=w297) -> ("States Out"=w296:string)  [unwired: 14 in]
      }
      frame "Action: Derive Inkscape Params" {
        # "Your code here.\n(You can make a copy of, or modify, this frame)"
        n113 = Unbundle By Name(w321) -> ("Main Image Params.Initial ScanSize"=w320:string, "Main Image Params.Initial XOffset"=w319:string, "Main Image Params.Initial YOffset"=w318:string, "Overlay Image Params.Initial ScanSize"=w317:string, "Overlay Image Params.Initial XOffset"=w316:string, "Overlay Image Params.Initial YOffset"=w315:string)
        n114 = Fract/Exp String To Number(string=w320) -> (number=w313:dbl)  [unwired: 3 in, 1 out]
        n115 = Fract/Exp String To Number(string=w319) -> (number=w312:dbl)  [unwired: 3 in, 1 out]
        n116 = Fract/Exp String To Number(string=w318) -> (number=w310:dbl)  [unwired: 3 in, 1 out]
        n117 = Fract/Exp String To Number(string=w317) -> (number=w299:dbl)  [unwired: 3 in, 1 out]
        n118 = Fract/Exp String To Number(string=w316) -> (number=w306:dbl)  [unwired: 3 in, 1 out]
        n119 = Fract/Exp String To Number(string=w315) -> (number=w307:dbl)  [unwired: 3 in, 1 out]
        n120 = Divide(x=w313, y=2.0) -> (x/y=w311:dbl)
        n121 = Divide(x=w299, y=2.0) -> (x/y=w309:dbl)
        n122 = Subtract(x=w311, y=w312) -> (x-y=w305:dbl)
        n123 = Add(x=w311, y=w310) -> (x+y=w303:dbl)
        n124 = Subtract(x=w309, y=w306) -> (x-y=w304:dbl)
        n125 = Add(x=w309, y=w307) -> (x+y=w302:dbl)
        n126 = Subtract(x=w305, y=w304) -> (x-y=w300:dbl)
        n127 = Subtract(x=w303, y=w302) -> (x-y=w301:dbl)
        n128 = Bundle(w300, w301, w299) -> (→"Inkscape Config":cluster{dbl, dbl, dbl})  [unwired: 1 in]
        n129 = call <vilib>:"Add State(s) to Queue__JKI_lib_State_Machine.vi"("State(s) in (\"\")"=w324) -> ("States Out"=w323:string)  [unwired: 14 in]
      }
    }
  }
  "Error Out" <- w1
